vi "8bit sync-Stitch cam video.vi"(6 "Initial frame":bool, 8 "error in (no error)":errorcluster, 9 "Resampled Cam video":T1, 10 "Input image":T1, 11 "Ctrl refs":T2) -> (0 "error out":errorcluster, 2 "Output image":T1)   [LabVIEW 2020]
uses:
  <vilib>/vision/Image Controls.llb/IMAQ Image.ctl
  Timelapse Viewer/Typedefs/8-bit video export window ctrl refs.ctl
  Typedefs/Bright-Contr-Gamma cluster.ctl
  Timelapse Viewer/Typedefs/Speed graph behaviour enum.ctl
  Functional Imaging Viewer/Typedefs/Get-Set-Clear Control.ctl
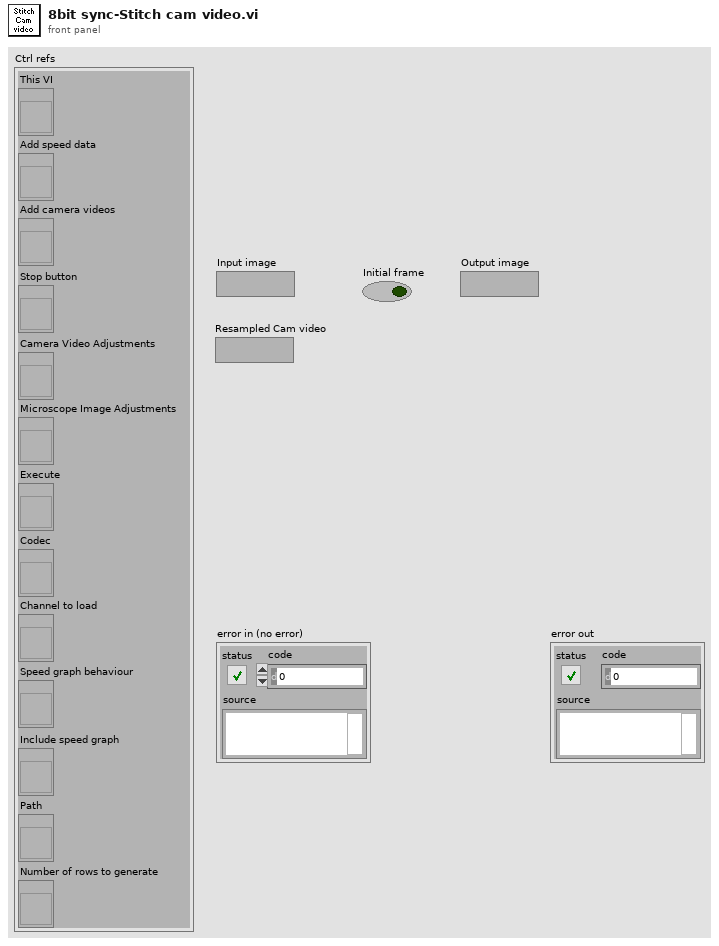
[diagram p1: front panel]
types:
  T1 = typedef "IMAQ Image.ctl" = refnum<image>
  T2 = typedef "8-bit video export window ctrl refs.ctl" = cluster{"This VI":refnum<vi>, "Add speed data":refnum<vi>, "Add camera videos":refnum<vi>, "Stop button":refnum<vi>, "Camera Video Adjustments":refnum<vi>, "Microscope Image Adjustments":refnum<vi>, "Execute":refnum<vi>, "Codec":refnum<vi>, "Channel to load":refnum<vi>, "Speed graph behaviour":refnum<vi>, "Include speed graph":refnum<vi>, "Number of rows to generate":refnum<vi>, "Path":refnum<vi>}
  T3 = enum16{"If Y mismatch then place near the top", "If Y mismatch then place near the bottom"}
  T4 = typedef "Get-Set-Clear Control.ctl" = enum16{"Get", "Set", "Clear"}
  T5 = typedef "Cam videos cluster.ctl" = cluster{"Vid 1":T1, "Vid 2":T1, "Vid 3":T1, "Vid 4":T1, "Vid1 Rel time (ms)":u32, "Vid2 Rel time (ms)":u32, "Vid3 Rel time (ms)":u32, "Vid4 Rel time (ms)":u32}
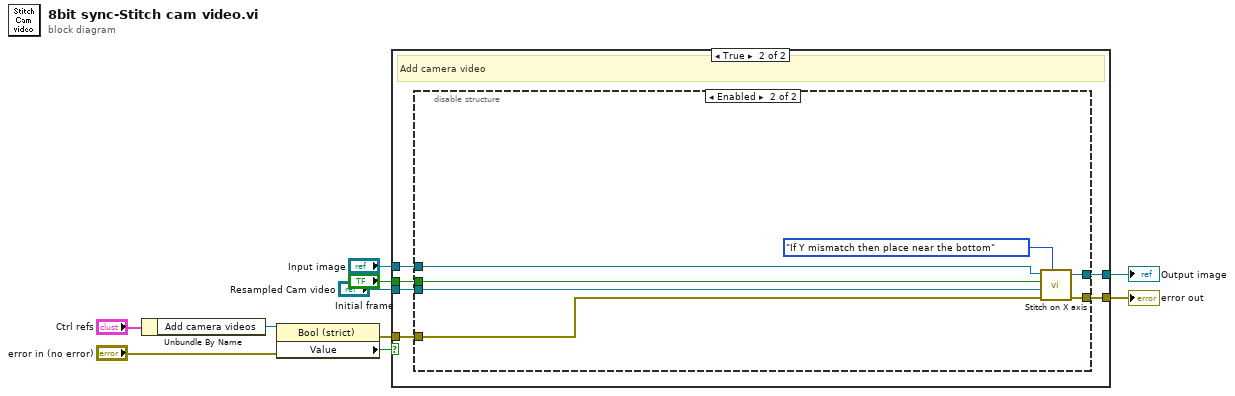
[diagram p0: block diagram]
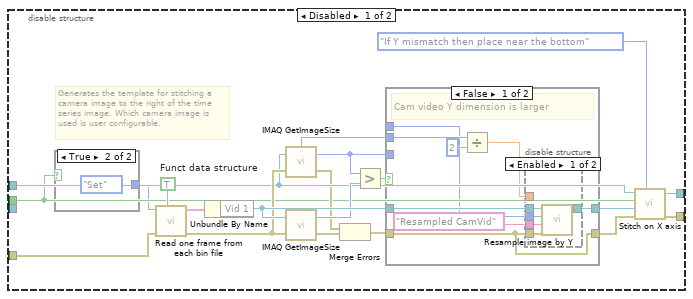
[diagram p3: hidden frame]
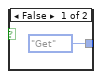
[diagram p4: hidden frame]
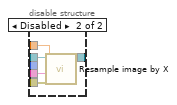
[diagram p5: hidden frame]
diagram:
  n1 = Unbundle By Name("Ctrl refs") -> ("Add camera videos"=w10:refnum<vi>)
  n2 = property class="Bool (strict)"(reference=w10, error in="error in (no error)") -> (error out=w8:errorcluster, "Value"=w9:bool)  [unwired: 1 out]
  n3 = case shown="True" w9 {
    tunnel: [w11 w17] -> w3
    tunnel: [w12 w18] -> w4
    tunnel: w8 -> [w12 w14]
    tunnel: "Initial frame" -> [_ w15]
    tunnel: "Input image" -> [w11 w16]
    tunnel: "Resampled Cam video" -> [_ w13]
    frame False {
      # "Do not add camera video"
    }
    frame True {
      # "Add camera video"
      n4 = disable-structure shown="Enabled" {
        disable-tunnel: [w40 w69] -> w18
        disable-tunnel: [w39 w68] -> w17
        disable-tunnel: w16 -> [w30 w67]
        disable-tunnel: w15 -> [w26 w66]
        disable-tunnel: w14 -> [w24 w63]
        disable-tunnel: w13 -> [_ w64]
        frame Disabled {
          w32 = TRUE  # Funct data structure
          # "Generates the template for stitching a camera image to the right of the time series image. Which camera image is used is user configurable."
          n5 = case shown="True" w26 {
            tunnel: [Get-Set-Clear_Control."Get" ("GEt set .bin refs") Get-Set-Clear_Control."Set" ("GEt set .bin refs")] -> w25
            frame False {
            }
            frame True {
            }
          }
          n6 = call "Read one frame from each bin file.vi"("Funct data structure"=w32, "error in (no error)"=w24, "Get/set"=w25) -> ("Error out"=w33:errorcluster, "Cam videos cluster"=w37:T5, "Master video's frame number (unity-based)"=w29:i32)  [unwired: 6 in]
          n7 = Unbundle By Name(w37) -> ("Vid 1"=w38:T1)
          n8 = call "IMAQ GetImageSize"("Image"=w30, "error in (no error)"=w33) -> ("Y Resolution"=w36:i32, "X Resolution"=w23:i32, "error out"=w28:errorcluster)  [unwired: 2 out]
          n9 = call "IMAQ GetImageSize"("Image"=w38, "error in (no error)"=w33) -> ("Y Resolution"=w34:i32, "error out"=w27:errorcluster)  [unwired: 3 out]
          n10 = Merge Errors(w28, w27) -> (w22:errorcluster)
          n11 = Greater?(x=w36, y=w34) -> (0:w35:bool)
          n12 = case shown="False" w35 {
            tunnel: w36 -> [_ _]
            tunnel: w38 -> [w50 w62]
            tunnel: [w48 w62] -> w31
            tunnel: w22 -> [w44 w61]
            tunnel: w23 -> [w47 _]
            tunnel: [w44 w61] -> w21
            tunnel: [w43 _] -> w19
            frame False {
              # "Cam video Y dimension is larger"
              n13 = Divide(x=w47, y=2) -> (x/y=w45:dbl)
              n14 = disable-structure shown="Enabled" {
                disable-tunnel: w50 -> [w55 w60]
                disable-tunnel: "Resampled CamVid" ("Resampled Image Name") -> [w54 w59]
                disable-tunnel: [w53 w58] -> w48
                disable-tunnel: w44 -> [w52 w57]
                disable-tunnel: w43 -> [w51 _]
                disable-tunnel: w45 -> [_ w56]
                frame Enabled {
                  n15 = call "Resample image by Y.vi"("error in (no error)"=w52, "Resampled Image Name"=w54, "Y Resolution"=w51, "Refnum in"=w55) -> ("Refnum out"=w53:T1)  [unwired: 7 in]
                }
                frame Disabled {
                  n16 = call "Resample image by X.vi"("error in (no error)"=w57, "Resampled Image Name"=w59, "X Resolution"=w56, "Refnum in"=w60) -> ("Refnum out"=w58:T1)  [unwired: 7 in]
                }
              }
            }
            frame True {
              # "Cam video Y dimension is smaller"
            }
          }
          n17 = call "Stitch on X axis.vi"("Enum"=T3."If Y mismatch then place near the bottom", "error in (no error)"=w21, "Right Video"=w31, "Initial frame"=w26, "Left Video"=w30) -> ("error out"=w40:errorcluster, "Resulting video"=w39:T1)  [unwired: 5 in]
        }
        frame Enabled {
          n18 = call "Stitch on X axis.vi"("Enum"=T3."If Y mismatch then place near the bottom", "error in (no error)"=w63, "Right Video"=w64, "Initial frame"=w66, "Left Video"=w67) -> ("error out"=w69:errorcluster, "Resulting video"=w68:T1)  [unwired: 5 in]
        }
      }
    }
  }
  "Output image" <- w3
  "error out" <- w4
